vi "Set Measurement Properties.vi"(6 "Auto Range":bool, 7 "Measurement Type":T1=10 items=["Continuity", "Current AC", "Current DC", "Diode", "Frequency", "Resistance 4-wire", "Period", "Resistance 2-wire", "Temperature", "Voltage AC", "Voltage DC", "Voltage DC Ratio", "Capacitance"], 8 "error in (no error)":errorcluster, 9 "Resolution":dbl=1e-06 format="%#_6e", 10 "Manual Range":dbl=1.0 format="%#_13g", 11 "3446X in":refnum<class "3446X.lvclass">) -> (0 "error out":errorcluster, 3 "3446X out":refnum<class "3446X.lvclass">)   [LabVIEW 2018]
uses:
  3446X.lvclass
  PPLs/DMM/Parent/DMM.lvlibp/Custom Controls/Measurement Type.ctl
  PPLs/DMM/Parent/DMM.lvlibp/DMM.lvclass
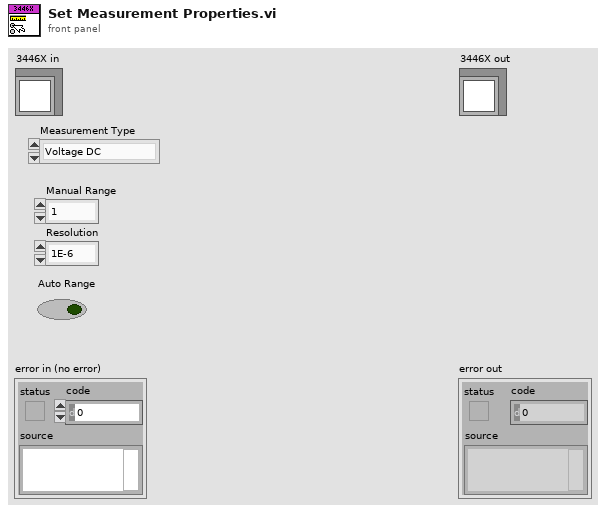
[diagram p1: front panel]
types:
  T1 = typedef "DMM.lvlibp/DMM.lvclass/Measurement Type.ctl" = u32
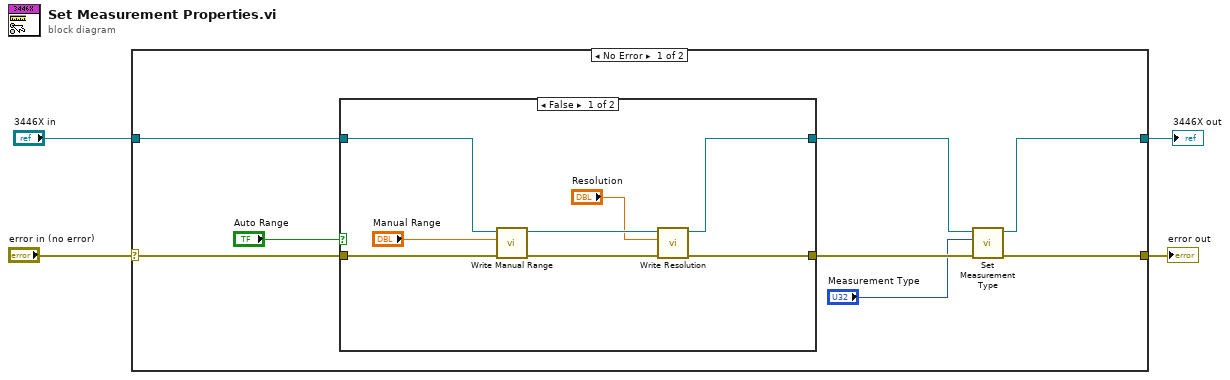
[diagram p0: block diagram]
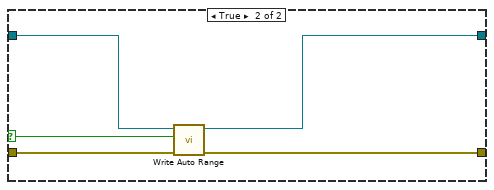
[diagram p2: hidden frame]
diagram:
  n1 = case shown="No Error" "error in (no error)" {
    selector: "error in (no error)" -> [w12 w27]
    tunnel: [w8 w27] -> w3
    tunnel: [w5 w26] -> w1
    tunnel: "3446X in" -> [w10 w26]
    frame No Error {
      n2 = case shown="False" "Auto Range" {
        selector: "Auto Range" -> [_ w24]
        tunnel: w12 -> [w20 w25]
        tunnel: w10 -> [w17 w23]
        tunnel: [w15 w22] -> w6
        tunnel: [w18 w21] -> w9
        frame False {
          n3 = call "Write Manual Range.vi"("error in (no error)"=w20, "Manual Range"="Manual Range", "3446X in"=w17) -> ("error out"=w19:errorcluster, "3446X out"=w16:refnum<class "3446X.lvclass">)  [unwired: 7 in]
          n4 = call "Write Resolution.vi"("error in (no error)"=w19, "Resolution"="Resolution", "3446X in"=w16) -> ("error out"=w18:errorcluster, "3446X out"=w15:refnum<class "3446X.lvclass">)  [unwired: 7 in]
        }
        frame True {
          n5 = call "Write Auto Range.vi"("error in (no error)"=w25, "Auto Range"=w24, "3446X in"=w23) -> ("error out"=w21:errorcluster, "3446X out"=w22:refnum<class "3446X.lvclass">)  [unwired: 7 in]
        }
      }
      n6 = call-dynamic "Set Measurement Type.vi"("error in (no error)"=w9, "Measurement Type"="Measurement Type", "3446X in"=w6) -> ("error out"=w8:errorcluster, "3446X out"=w5:refnum<class "3446X.lvclass">)  [unwired: 7 in]
    }
    frame Error {
    }
  }
  "error out" <- w3
  "3446X out" <- w1
